vi "(백업)setup complete.vi"   [LabVIEW 2014]
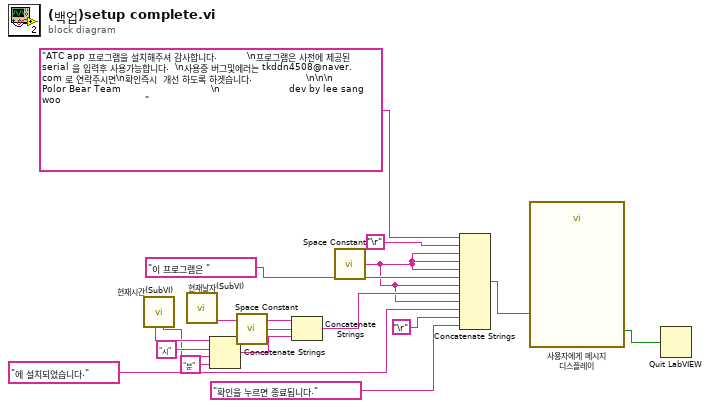
[diagram p0: block diagram]
diagram:
  n1 = call "현재시간(SubVI).vi"() -> ("분 문자열"=w15:string, "시 문자열"=w17:string)  [unwired: 3 in, 7 out]
  n2 = call "현재날자(SubVI).vi"() -> ("월,일 을 문자열로"=w11:string)  [unwired: 5 in, 6 out]
  n3 = Concatenate Strings(w17, "시", w15, "분" ("문자열")) -> (w13:string)
  n4 = call <vilib>:"Space Constant.vi"() -> ("String"=w12:string)
  n5 = Concatenate Strings(w11, w12, w13) -> (w7:string)
  n6 = call <vilib>:"Space Constant.vi"() -> ("String"=w6:string)
  n7 = Concatenate Strings("ATC app 프로그램을 설치해주셔 감사합니다.          \n프로그램은 사전에 제공된 serial 을 입력후 사용가능합니다.  \n사용중 버그및에러는 tkddn4508@naver.com 로 연락주시면\n확인즉시  개선 하도록 하겟습니다.                  \n\n\n                           Polor Bear Team                              \n                       dev by lee sang woo                            " ("Message"), "\r", w6, w6, w6, "이 프로그램은 ", w6, w7, w6, "에 설치되었습니다.", "\r", "확인을 누르면 종료됩니다.") -> (w2:string)
  n8 = call "사용자에게 메시지 디스플레이"("Message"=w2) -> ("닫기"=w1:bool)  [unwired: 9 in, 1 out]
  n9 = Quit LabVIEW(quit? (T)=w1) -> ()
